vi "Array To List.vi"(11 "Array":string[](array[string])) -> (3 "String":string)   [LabVIEW 2016, in "JSON Value.lvclass"]
doc: "Converts an array of strings in to a comma separated list."
uses:
  JSON Value.lvclass
  <vilib>/Utility/error.llb/whitespace.ctl
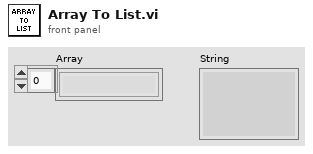
[diagram p1: front panel]
types:
  T1 = typedef "whitespace.ctl" = u16
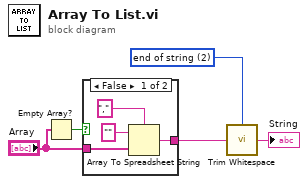
[diagram p0: block diagram]
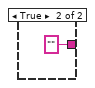
[diagram p2: hidden frame]
diagram:
  w1 = T1 2 items=["both", "start of string", "end of string"] ("location (both)")
  n1 = Empty Array?(array="Array") -> (empty?=w4:bool)
  n2 = case shown="False" w4 {
    tunnel: [w6 "" ("spreadsheet string")] -> w3
    tunnel: "Array" -> [w9 _]
    frame False {
      n3 = Array To Spreadsheet String(delimiter (Tab)=",", array=w9, 3:"" ("format string")) -> (spreadsheet string=w6:string)
    }
    frame True {
    }
  }
  n4 = call <vilib>:"Trim Whitespace.vi"("string"=w3, "location (both)"=w1) -> ("trimmed string"=→"String":string)
